vi "송신.vi"() -> ()   [LabVIEW 2014]
uses:
  <vilib>/Analysis/NI_AALBase.lvlib
panel:
  in  "정지":bool
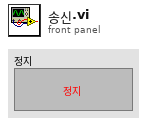
[diagram p1: front panel]
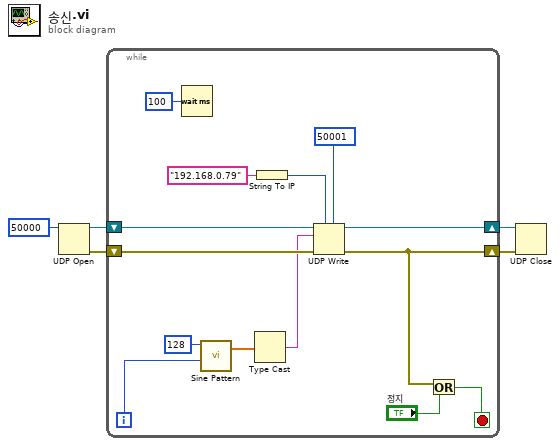
[diagram p0: block diagram]
diagram:
  n1 = UDP Open(11:u16 50000 ("포트")) -> (port=w5:refnum<k16>, 0:w3:errorcluster)  [unwired: 4 in, 1 out]
  n2 = while {
    shift-right: [w18] -> w4
    shift-left: w5 -> [w19]
    shift-right: [w12] -> w2
    shift-left: w3 -> [w17]
    i -> [w9]
    stop <- w11 stop-if-true
    n3 = Wait (ms)(milliseconds to wait=u32 100 ("대기 시간(ms)")) -> ()  [unwired: 1 out]
    n4 = call <vilib>:"Sine Pattern.vi"("phase(degrees)"=w9, "samples"=128) -> ("Sinusoidal Pattern"=w7:dbl[])  [unwired: 2 in, 1 out]
    n5 = Type Cast(x=w7) -> (*(type *) &x=w6:string)  [unwired: 1 in]
    n6 = String To IP(1:"192.168.0.79" ("이름")) -> (0:w16:u32)
    n7 = UDP Write(address=w16, port or service name=u16 50001 ("포트 또는 서비스 이름"), connection ID=w19, data in=w6, 8:w17) -> (error out=w12:errorcluster, 3:w18:refnum<k16>)  [unwired: 1 in]
    n8 = Or(x=w12, y="정지") -> (x .or. y?=w11:bool)
  }
  n9 = UDP Close(connection ID=w4, 8:w2) -> ()  [unwired: 2 out]
